vi "Uneven Derivative.vi"() -> ()   [LabVIEW 2023]
uses:
  <vilib>/express/express arith-compare/Formula/XNode/ExpressFormulaBlockNode.xnode
panel:
  out "XY Graph 2":cluster{dbl[], dbl[]}(graph)
  out "XY Graph":cluster{dbl[], dbl[]}(graph)
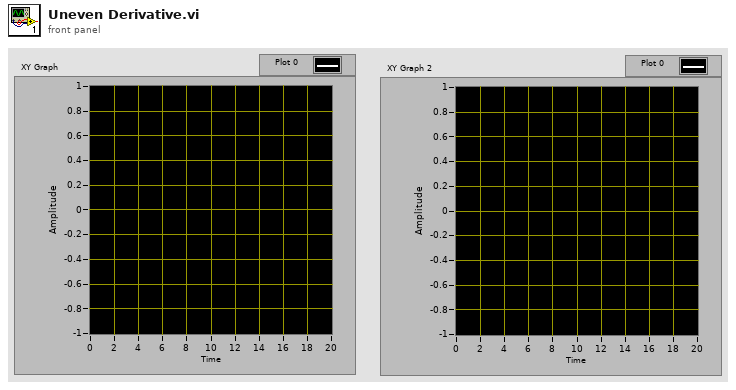
[diagram p1: front panel]
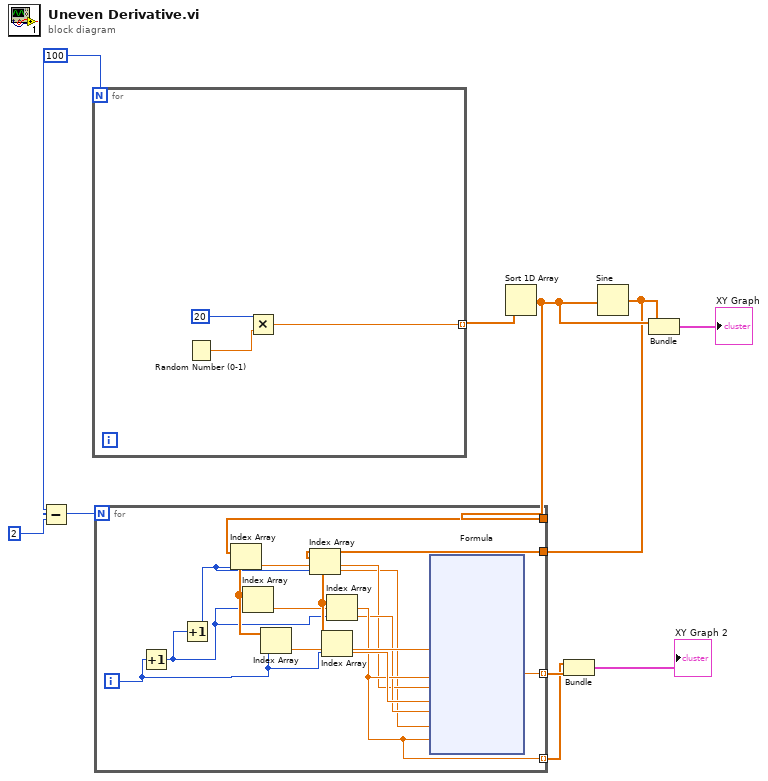
[diagram p0: block diagram]
diagram:
  w6 = 100
  n1 = Subtract(x=w6, y=2) -> (x-y=w7:i32)
  n2 = for {
    N: w6 -> [_]
    tunnel: [w11] -> w10 mode=indexing
    n3 = Random Number (0-1)() -> (number: 0 to 1=w13:dbl)
    n4 = Multiply(x=20, y=w13) -> (x*y=w11:dbl)
  }
  n5 = Sort 1D Array(array=w10) -> (sorted array=w5:dbl[])
  n6 = Sine(x=w5) -> (sin(x)=w4:dbl[])
  n7 = for {
    N: w7 -> [_]
    tunnel: w5 -> [w25]
    tunnel: w4 -> [w23]
    tunnel: [w21] -> w3 mode=indexing
    tunnel: [w17] -> w1 mode=indexing
    i -> [w22]
    n8 = Increment(x=w22) -> (x+1=w20:i32)
    n9 = Increment(x=w20) -> (x+1=w24:i32)
    n10 = Index Array(array=w25, index=w24) -> (element=w15:dbl)
    n11 = Index Array(array=w25, index=w20) -> (element=w17:dbl)
    n12 = Index Array(array=w25, index=w22) -> (element=w19:dbl)
    n13 = Index Array(array=w23, index=w24) -> (element=w14:dbl)
    n14 = Index Array(array=w23, index=w22) -> (element=w18:dbl)
    n15 = Index Array(array=w23, index=w20) -> (element=w16:dbl)
    n16 = xnode "Formula"("X1"=w19, "X2"=w17, "X3"=w15, "Y1"=w18, "Y2"=w16, "Y3"=w14, "X"=w17) -> ("Result"=w21:dbl)  [unwired: 1 in, 1 out]
  }
  n17 = Bundle(w1, w3) -> (→"XY Graph 2":cluster{dbl[], dbl[]})  [unwired: 1 in]
  n18 = Bundle(w5, w4) -> (→"XY Graph":cluster{dbl[], dbl[]})  [unwired: 1 in]
